vi "DAQmx System Info.vi"() -> ()   [LabVIEW 2018]
uses:
  <resource>/objmgr/daqmx.rc
panel:
  in  "error in (no error)":errorcluster
  out "error out":errorcluster
  out "NI-DAQmx Device Information":string
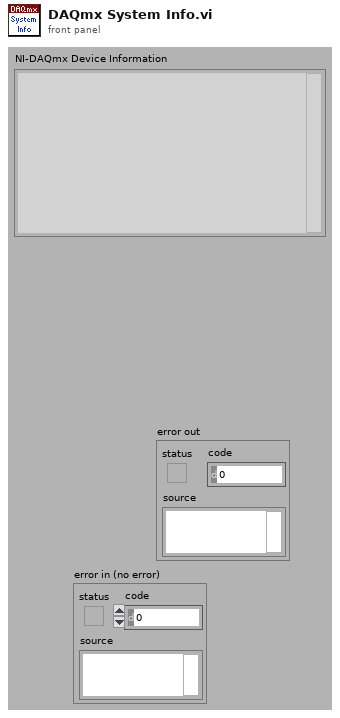
[diagram p1: front panel]
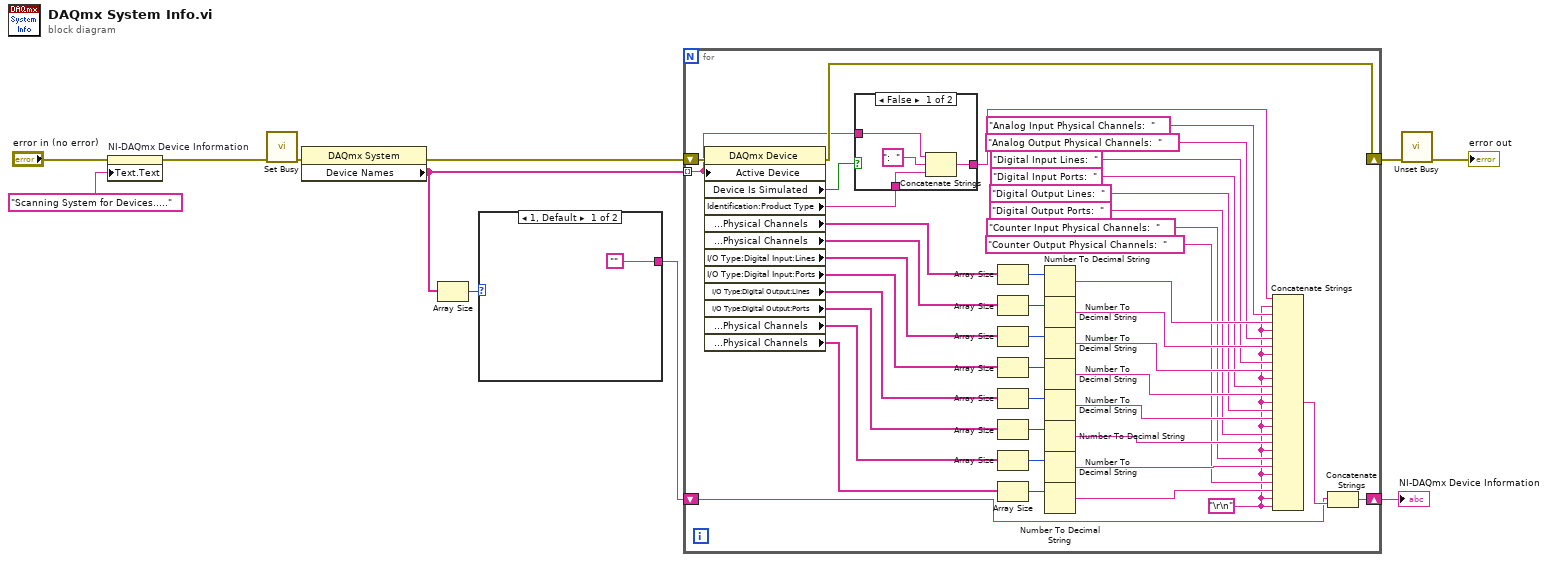
[diagram p0: block diagram]
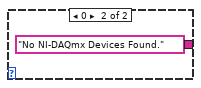
[diagram p2: hidden frame]
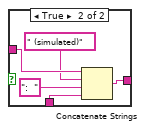
[diagram p3: hidden frame]
diagram:
  n1 = property on="NI-DAQmx Device Information" class="Str"(error in="error in (no error)", "Text.Text"="Scanning System for Devices.....") -> (error out=w9:errorcluster)  [unwired: 1 in, 1 out]
  n2 = call <vilib>:"Set Busy.vi"("error in (no error)"=w9) -> ("error out"=w8:errorcluster)  [unwired: 9 in, 1 out]
  n3 = property class="DAQmx System"(error in=w8) -> (error out=w10:errorcluster, "Device Names"=w4:tag[])  [unwired: 1 in, 1 out]
  n4 = Array Size(array=w4) -> (size(s)=w5:i32)
  n5 = case shown="1, Default" w5 {
    tunnel: ["" "No NI-DAQmx Devices Found."] -> w3
    frame 1, Default {
    }
    frame 0 {
    }
  }
  n6 = for {
    tunnel: w4 -> [w14] mode=indexing
    shift-right: [w55] -> w11
    shift-left: w3 -> [w22]
    shift-right: [w18] -> w2
    shift-left: w10 -> [w19]
    w20 = "\r\n"
    n7 = property class="DAQmx Device"(error in=w19, "Active Device"=w14) -> (error out=w18:errorcluster, "Device Is Simulated"=w17:bool, "Identification:Product Type"=w16:string, "I/O Type:Analog Input:Physical Channels"=w54:tag[], "I/O Type:Analog Output:Physical Channels"=w47:tag[], "I/O Type:Digital Input:Lines"=w42:tag[], "I/O Type:Digital Input:Ports"=w41:tag[], "I/O Type:Digital Output:Lines"=w40:tag[], "I/O Type:Digital Output:Ports"=w39:tag[], "I/O Type:Counter Input:Physical Channels"=w38:tag[], "I/O Type:Counter Output:Physical Channels"=w36:tag[])  [unwired: 1 in, 1 out]
    n8 = case shown="False" w17 {
      tunnel: w16 -> [w57 w60]
      tunnel: [w58 w64] -> w15
      tunnel: w14 -> [w59 w63]
      frame False {
        n9 = Concatenate Strings(w59, ":  " ("string"), w57) -> (w58:string)
      }
      frame True {
        n10 = Concatenate Strings(w63, " (simulated)" ("string"), ":  " ("string"), w60) -> (w64:string)
      }
    }
    n11 = Array Size(array=w54) -> (size(s)=w53:i32)
    n12 = Array Size(array=w47) -> (size(s)=w48:i32)
    n13 = Array Size(array=w42) -> (size(s)=w49:i32)
    n14 = Array Size(array=w41) -> (size(s)=w46:i32)
    n15 = Array Size(array=w40) -> (size(s)=w45:i32)
    n16 = Array Size(array=w39) -> (size(s)=w44:i32)
    n17 = Array Size(array=w38) -> (size(s)=w43:i32)
    n18 = Array Size(array=w36) -> (size(s)=w37:i32)
    n19 = Number To Decimal String(number=w53) -> (decimal integer string=w50:string)  [unwired: 1 in]
    n20 = Number To Decimal String(number=w48) -> (decimal integer string=w34:string)  [unwired: 1 in]
    n21 = Number To Decimal String(number=w49) -> (decimal integer string=w32:string)  [unwired: 1 in]
    n22 = Number To Decimal String(number=w46) -> (decimal integer string=w30:string)  [unwired: 1 in]
    n23 = Number To Decimal String(number=w45) -> (decimal integer string=w28:string)  [unwired: 1 in]
    n24 = Number To Decimal String(number=w44) -> (decimal integer string=w26:string)  [unwired: 1 in]
    n25 = Number To Decimal String(number=w43) -> (decimal integer string=w24:string)  [unwired: 1 in]
    n26 = Number To Decimal String(number=w37) -> (decimal integer string=w23:string)  [unwired: 1 in]
    n27 = Concatenate Strings(w15, w20, "Analog Input Physical Channels:  ", w50, w20, "Analog Output Physical Channels:  ", w34, w20, "Digital Input Lines:  ", w32, w20, "Digital Input Ports:  ", w30, w20, "Digital Output Lines:  ", w28, w20, "Digital Output Ports:  ", w26, w20, "Counter Input Physical Channels:  ", w24, w20, "Counter Output Physical Channels:  ", w23, w20, w20) -> (w52:string)
    n28 = Concatenate Strings(w22, w52) -> (w55:string)
  }
  "NI-DAQmx Device Information" <- w11
  n29 = call <vilib>:"Unset Busy.vi"("error in (no error)"=w2) -> ("error out"=→"error out":errorcluster)  [unwired: 10 in]
